vi "Digital_write.vi"(10 "Milliseconds to wait":u32, 11 "lines":tag) -> ()   [LabVIEW 2020]
uses:
  <vilib>/DAQmx/write.llb/DAQmx Write (Digital Bool 1Line 1Point).vi
  <vilib>/DAQmx/create/channels.llb/DAQmx Create Channel (DO-Digital Output).vi
  <vilib>/DAQmx/miscellaneous.llb/DAQmx Fill In Error Info.vi
panel:
  in  "y":bool
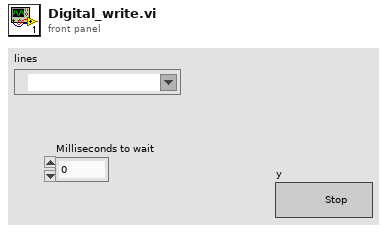
[diagram p1: front panel]
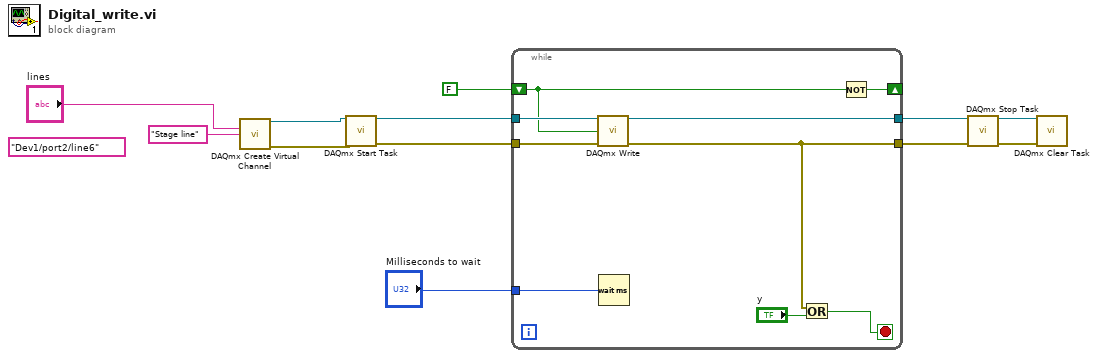
[diagram p0: block diagram]
diagram:
  (unwired) tag "Dev1/port2/line6" ("lines")
  n1 = call-poly <vilib>:"DAQmx Create Virtual Channel.vi"("lines"="lines", "name to assign"="Stage line") -> ("task out"=w10:refnum<k21>, "error out"=w9:errorcluster)  [unwired: 12 in]
  n2 = call <vilib>:"DAQmx Start Task.vi"("task/channels in"=w10, "error in"=w9) -> ("task out"=w12:refnum<k21>, "error out"=w11:errorcluster)  [unwired: 12 in]
  n3 = while {
    tunnel: w12 -> [w21]
    tunnel: w11 -> [w20]
    shift-right: [w19] -> _
    shift-left: FALSE ("data") -> [w18]
    tunnel: [w17] -> w7
    tunnel: [w14] -> w6
    tunnel: "Milliseconds to wait" -> [w13]
    stop <- w16 stop-if-true
    n4 = call-poly <vilib>:"DAQmx Write.vi"("task/channels in"=w21, "data"=w18, "error in"=w20) -> ("task out"=w17:refnum<k21>, "error out"=w14:errorcluster)  [unwired: 10 in, 1 out]
    n5 = Wait (ms)(milliseconds to wait=w13) -> ()  [unwired: 1 out]
    n6 = Or(x=w14, y="y") -> (x .or. y?=w16:bool)
    n7 = Not(x=w18) -> (.not. x?=w19:bool)
  }
  n8 = call <vilib>:"DAQmx Stop Task.vi"("task/channels in"=w7, "error in"=w6) -> ("task out"=w5:refnum<k21>, "error out"=w4:errorcluster)  [unwired: 12 in]
  n9 = call <vilib>:"DAQmx Clear Task.vi"("task in"=w5, "error in"=w4) -> ()  [unwired: 13 in, 1 out]
